vi "Send UNREGISTER.vi"(8 "error in (no error)":errorcluster, 9 "Unregister Request":T1, 10 "Message loop data (in)":T2, 11 "WAMP Client in":refnum<class "WAMP Client.lvclass">) -> (0 "error out":errorcluster, 2 "Message loop data (out)":T2, 3 "WAMP Client out":refnum<class "WAMP Client.lvclass">)   [LabVIEW 2020, in "wamplv.lvlib" / "WAMP Client.lvclass"]
uses:
  WAMP Client.lvclass
  TypeDef/Message Loop Shift Reg Data.ctl
  TypeDef/REGISTER Request Data.ctl
  TypeDef/Success or error.ctl
  API/TypeDefs/Combined error.ctl
  API/TypeDefs/WAMP error.ctl
  TypeDef/Publish Requests Map.ctl
  TypeDef/PUBLISH Request Data.ctl
  TypeDef/PUBLISH result.ctl
  TypeDef/Endpoint Data.ctl
  TypeDef/CALL Request Map.ctl
  TypeDef/CALL Request Data.ctl
  API/TypeDefs/RESULT payload.ctl
  TypeDef/SUBSCRIBE Requests Map.ctl
  TypeDef/SUBSCRIBE Request Data.ctl
  TypeDef/Subscribe Result.ctl
  TypeDef/EVENT payload.ctl
  TypeDef/Subscriptions Map.ctl
  TypeDef/Subscription Details.ctl
  TypeDef/Unsubscribe Requests Map.ctl
  TypeDef/UNSUBSCRIBE Request Data.ctl
  TypeDef/UNSUBSCRIBE Result.ctl
  TypeDef/Unregister requests map.ctl
  TypeDef/Unregister request.ctl
  WAMP Client.lvclass/WAMP Client.ctl
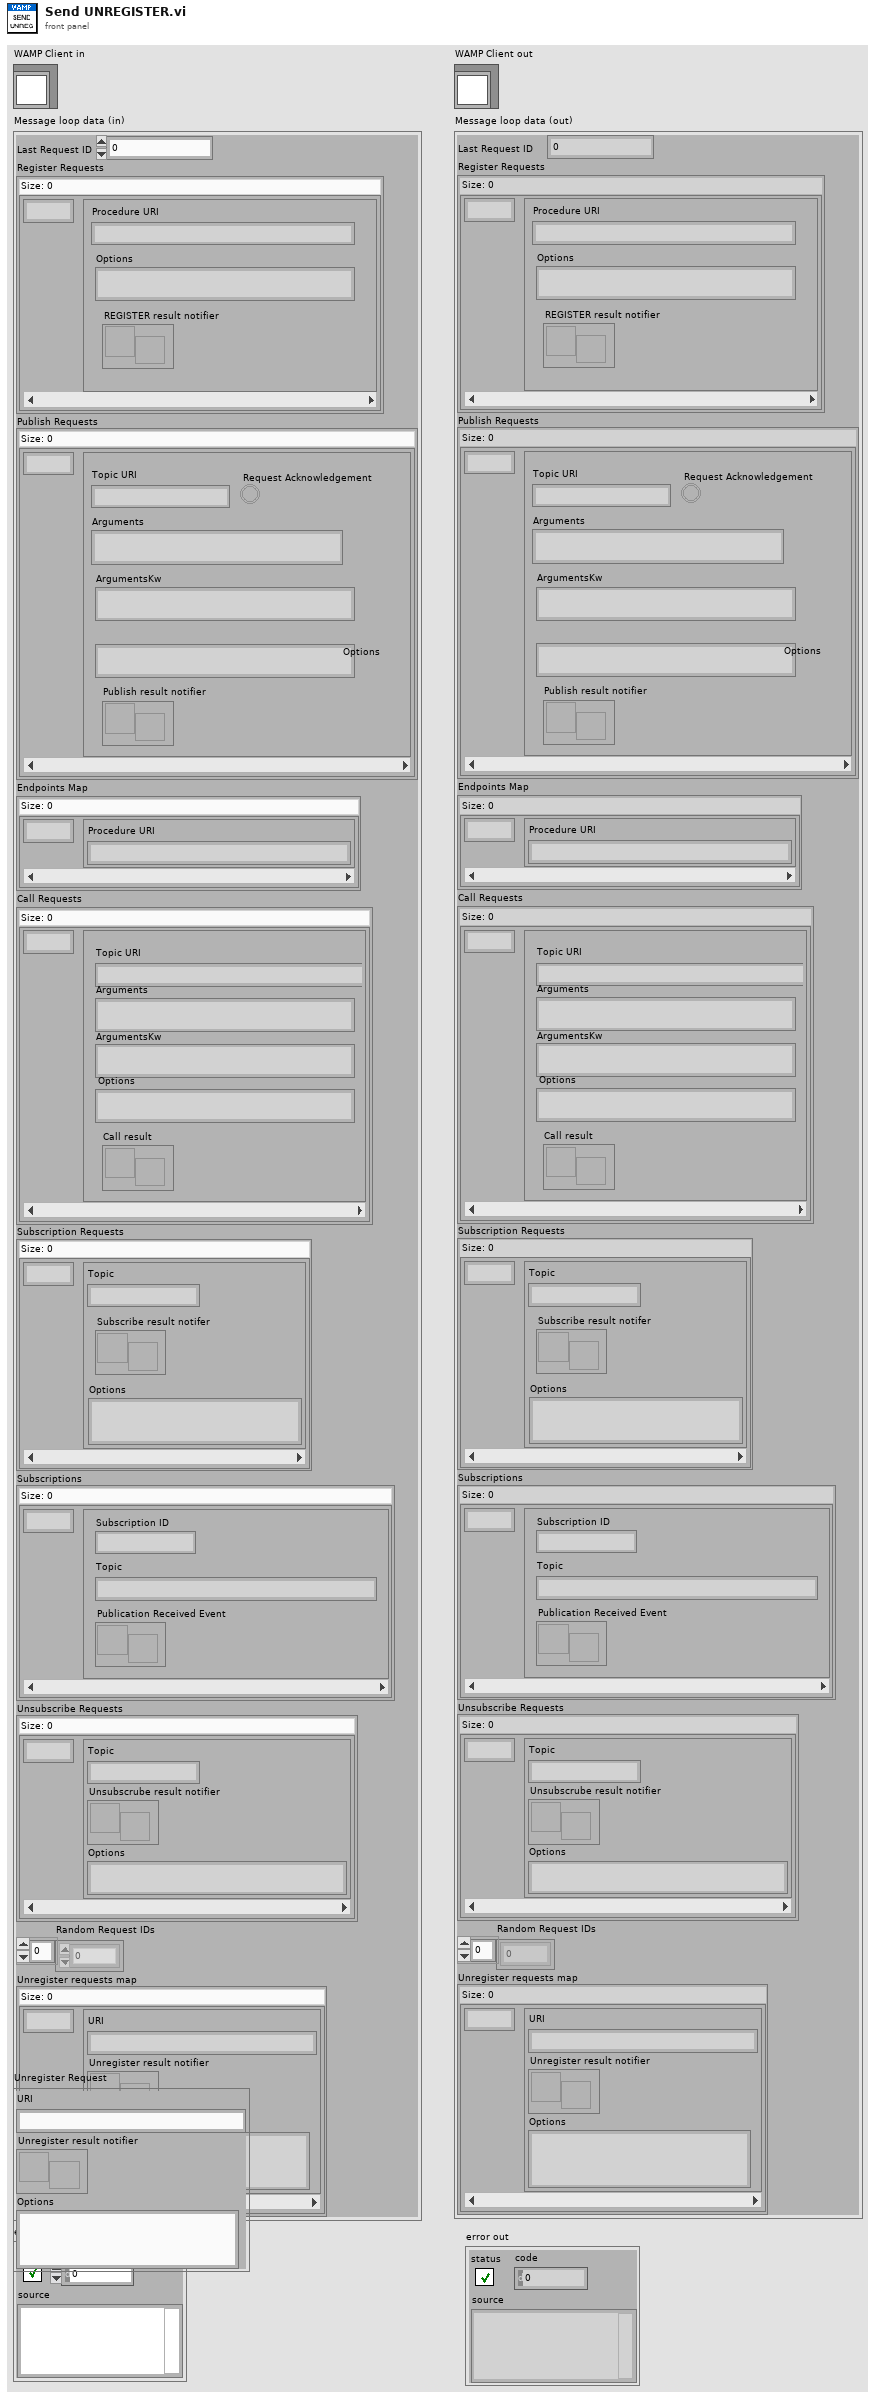
[diagram p1: front panel]
types:
  T1 = typedef "wamplv.lvlib/WAMP Client.lvclass/Unregister request.ctl" = cluster{"URI":string, "Unregister result notifier":refnum<notifier>, "Options":string}
  T2 = typedef "wamplv.lvlib/WAMP Client.lvclass/Message Loop Shift Reg Data.ctl" = cluster{"Last Request ID":u64, "Register Requests":map{u64, T3}, "Publish Requests":T4, "Endpoints Map":map{u64, T6}, "Call Requests":T7, "Subscription Requests":T9, "Subscriptions":T11, "Unsubscribe Requests":T13, "Random Request IDs":u64[], "Unregister requests map":T15}
  T3 = typedef "wamplv.lvlib/WAMP Client.lvclass/REGISTER Request Data.ctl" = cluster{"Procedure URI":string, "Options":string, "REGISTER result notifier":refnum<notifier>}
  T4 = typedef "wamplv.lvlib/WAMP Client.lvclass/Publish Requests Map.ctl" = map{u64, T5}
  T5 = typedef "wamplv.lvlib/WAMP Client.lvclass/PUBLISH Request Data.ctl" = cluster{"Topic URI":string, "Arguments":string, "ArgumentsKw":string, "Request Acknowledgement":bool, "Options":string, "Publish result notifier":refnum<notifier>}
  T6 = typedef "wamplv.lvlib/WAMP Client.lvclass/Endpoint Data.ctl" = cluster{"Procedure URI":string}
  T7 = typedef "wamplv.lvlib/WAMP Client.lvclass/CALL Request Map.ctl" = map{u64, T8}
  T8 = typedef "wamplv.lvlib/WAMP Client.lvclass/CALL Request Data.ctl" = cluster{"Topic URI":string, "Arguments":string, "ArgumentsKw":string, "Options":string, "Call result":refnum<notifier>}
  T9 = typedef "wamplv.lvlib/WAMP Client.lvclass/SUBSCRIBE Requests Map.ctl" = map{u64, T10}
  T10 = typedef "wamplv.lvlib/WAMP Client.lvclass/SUBSCRIBE Request Data.ctl" = cluster{"Topic":string, "Subscribe result notifer":refnum<notifier>, "Options":string}
  T11 = typedef "wamplv.lvlib/WAMP Client.lvclass/Subscriptions Map.ctl" = map{u64, T12}
  T12 = typedef "wamplv.lvlib/WAMP Client.lvclass/Subscription Details.ctl" = cluster{"Subscription ID":u64, "Topic":string, "Publication Received Event":refnum<user-event>}
  T13 = typedef "wamplv.lvlib/WAMP Client.lvclass/Unsubscribe Requests Map.ctl" = map{u64, T14}
  T14 = typedef "wamplv.lvlib/WAMP Client.lvclass/UNSUBSCRIBE Request Data.ctl" = cluster{"Topic":string, "Unsubscrube result notifier":refnum<notifier>, "Options":string}
  T15 = typedef "wamplv.lvlib/WAMP Client.lvclass/Unregister requests map.ctl" = map{u64, T1}
  T16 = typedef "wamplv.lvlib/WAMP Client.lvclass/Success or error.ctl" = cluster{"Success?":bool, "URI":string, "Combined Error":T17}
  T17 = typedef "wamplv.lvlib/WAMP Client.lvclass/Combined error.ctl" = cluster{"Error?":bool, "WAMP Error":T18, "Error":errorcluster}
  T18 = typedef "wamplv.lvlib/WAMP Client.lvclass/WAMP error.ctl" = cluster{"Details":string, "ArgumentKw Payload":string, "Error?":bool, "Error URI":string, "Arguments Payload":string}
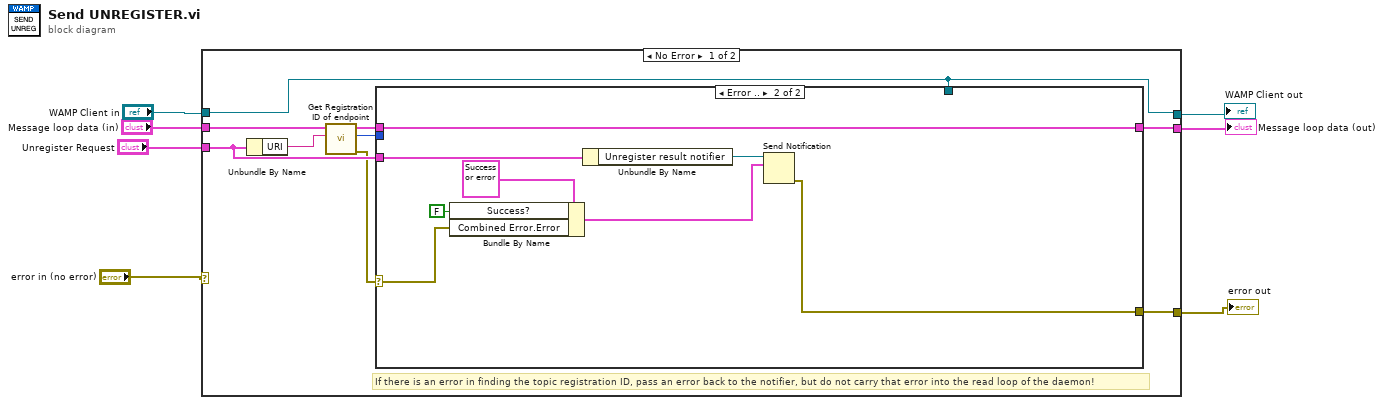
[diagram p0: block diagram]
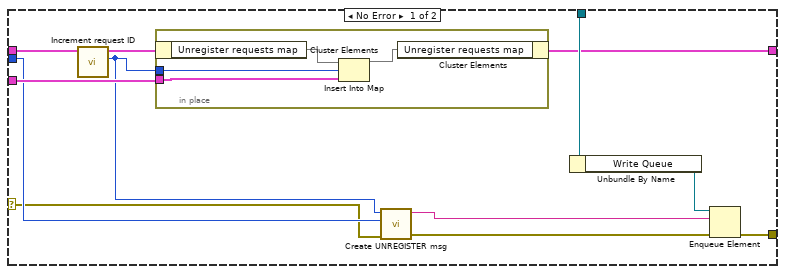
[diagram p2: hidden frame]
diagram:
  n1 = case shown="No Error" "error in (no error)" {
    selector: "error in (no error)" -> [_ w43]
    tunnel: [w15 w43] -> w6
    tunnel: [w16 w42] -> w4
    tunnel: "WAMP Client in" -> [w16 w42]
    tunnel: "Unregister Request" -> [w14 _]
    tunnel: "Message loop data (in)" -> [w13 w41]
    tunnel: [w8 w41] -> w2
    frame No Error {
      # "If there is an error in finding the topic registration ID, pass an error back to the notifier, but do not carry that error into the read loop of the daemon!"
      n2 = Unbundle By Name(w14) -> ("URI"=w11:string)
      n3 = call "Get Registration ID of endpoint.vi"("Endpoint URI"=w11, "Message loop data (in)"=w13) -> ("error out"=w9:errorcluster, "Registrtion ID"=w10:u64, "Message loop data (out)"=w12:T2)  [unwired: 7 in]
      n4 = case shown="Error .." w9 {
        selector: w9 -> [w19 w36]
        tunnel: w16 -> [w26 _]
        tunnel: [w25 w34] -> w15
        tunnel: w14 -> [w23 w40]
        tunnel: w12 -> [w21 w39]
        tunnel: w10 -> [w20 _]
        tunnel: [w17 w39] -> w8
        frame No Error {
          n5 = call "Increment request ID.vi"("Message Loop Shift Register Data (in)"=w21) -> ("New Request ID"=w22:u64, "Message Loop Shift Register Data (out)"=w18:T2)  [unwired: 9 in]
          n6 = in-place "In Place Element Structure" {
            in-place-border: w23 -> [w29]
            in-place-border: w22 -> [w30]
            n7 = in-place-cluster #1(w18) -> ("Unregister requests map"=w32:T15)
            n8 = Insert Into Map(map in=w32, key=w30, value=w29) -> (map out=w31:T15)  [unwired: 2 out]
            n9 = in-place-cluster #1("Unregister requests map"=w31) -> (w17:T2)
          }
          n10 = call "Create UNREGISTER msg.vi"("error in (no error)"=w19, "Registration ID"=w20, "Request ID"=w22) -> ("error out"=w28:errorcluster, "WAMP Message"=w27:string)  [unwired: 7 in]
          n11 = Unbundle By Name(w26) -> ("Write Queue"=w24:refnum<queue>)
          n12 = Enqueue Element(queue=w24, element=w27, error in (no error)=w28) -> (error out=w25:errorcluster)  [unwired: 1 in, 2 out]
        }
        frame Error {
          n13 = Bundle By Name(cluster=T16 {"Success?"=FALSE, "URI"="", "Combined Error"={"Error?"=FALSE, "WAMP Error"={"Details"="{}", "ArgumentKw Payload"="{}", "Error?"=FALSE, "Error URI"="", "Arguments Payload"=""}, "Error"={"status"=FALSE, "code"=0, "source"=""}}} ("notification"), "Success?"=FALSE, "Combined Error.Error"=w36) -> (w35:T16)
          n14 = Unbundle By Name(w40) -> ("Unregister result notifier"=w38:refnum<notifier>)
          n15 = Send Notification(notification=w35, notifier=w38) -> (error out=w34:errorcluster)  [unwired: 1 in, 1 out]
        }
      }
    }
    frame Error {
    }
  }
  "error out" <- w6
  "WAMP Client out" <- w4
  "Message loop data (out)" <- w2
